vi "Write minutesArc.vi"(8 "error in (no error)":errorcluster, 10 "minutesArc":dbl[unit] min=0.0 max=0.017453292519943295, 11 "Azimuth in":refnum<class "Azimuth.lvclass">) -> (0 "error out":errorcluster, 3 "Azimuth out":refnum<class "Azimuth.lvclass">)   [LabVIEW 2022 SP3, in "TCSDataDefinitions.lvlib" / "TCSCommand.lvlib" / "TargetConfiguration.lvlib" / "Target.lvlib" / "FixedTarget.lvlib" / "Azimuth.lvclass"]
uses:
  Azimuth.lvclass
  Azimuth.lvclass/Azimuth.ctl
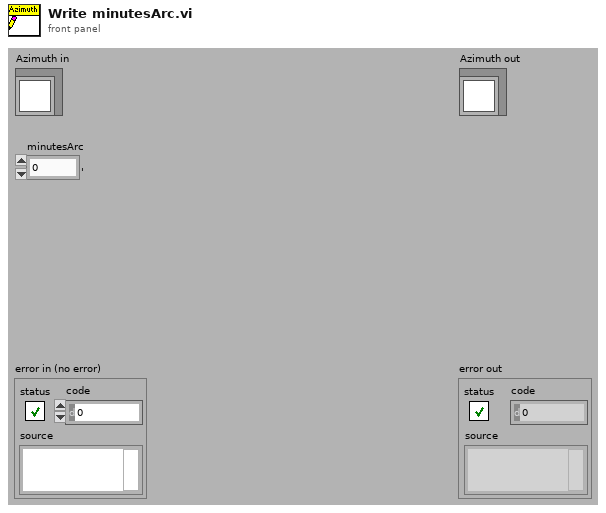
[diagram p1: front panel]
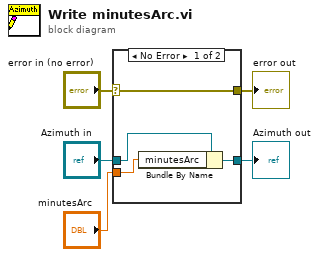
[diagram p0: block diagram]
diagram:
  n1 = case shown="No Error" "error in (no error)" {
    selector: "error in (no error)" -> [w9 w10]
    tunnel: [w9 w10] -> w4
    tunnel: [w7 w11] -> w2
    tunnel: "Azimuth in" -> [w8 w11]
    tunnel: "minutesArc" -> [w6 _]
    frame No Error {
      n2 = Bundle By Name(cluster=w8, "minutesArc"=w6) -> (w7:refnum<class "Azimuth.lvclass">)
    }
    frame Error {
    }
  }
  "error out" <- w4
  "Azimuth out" <- w2
